vi "TRANSPOSED_VERTREAD_CSV_import_control_lasers_and_SMs_and_ICC4C_CAM_Trigger.vi"() -> ()   [LabVIEW 2021]
uses:
  <vilib>/DAQmx/write.llb/DAQmx Write (Analog 1D DBL NChan 1Samp).vi
  <vilib>/DAQmx/create/channels.llb/DAQmx Create Channel (AO-Voltage-Basic).vi
  <vilib>/Utility/file.llb/Read Delimited Spreadsheet (DBL).vi
  <vilib>/DAQmx/miscellaneous.llb/DAQmx Fill In Error Info.vi
panel:
  out "Raw  Inner Loop Iternation":dbl
  out "Numeric":dbl
  out "Trigger_Phase_Iterations":i32
  out "Cam_Trigger_Lo":dbl
  out "Cam_Trigger_Hi":dbl
  out "Sequence Length":i32
  in  "Delay (ADDS 50ms)":i32
  in  "ICC4C 3 (0-10V)":dbl
  in  "ICC4C 2 (0-10V)":dbl
  in  "ICC4C 1 (0-10V)":dbl
  in  "ICC4C 0 (0-10V)":dbl
  in  "Y2 (-10-10V)":dbl
  in  "X2 (-10-10V)":dbl
  in  "Continue Cycle?":bool
  out "Full Cycles":i32
  out "Mirror_Phase_Iterations":i32
  out "Y1 (-10-10V)":dbl format="%_6g"
  out "X1 (-10-10V)":dbl format="%_6g"
  in  "Blanking (0-10v)":dbl=10.0
  in  "561 (0-10v)":dbl
  in  "514 (0-10v)":dbl
  in  "488 (0-10v)":dbl
  in  "445 (0-10v)":dbl
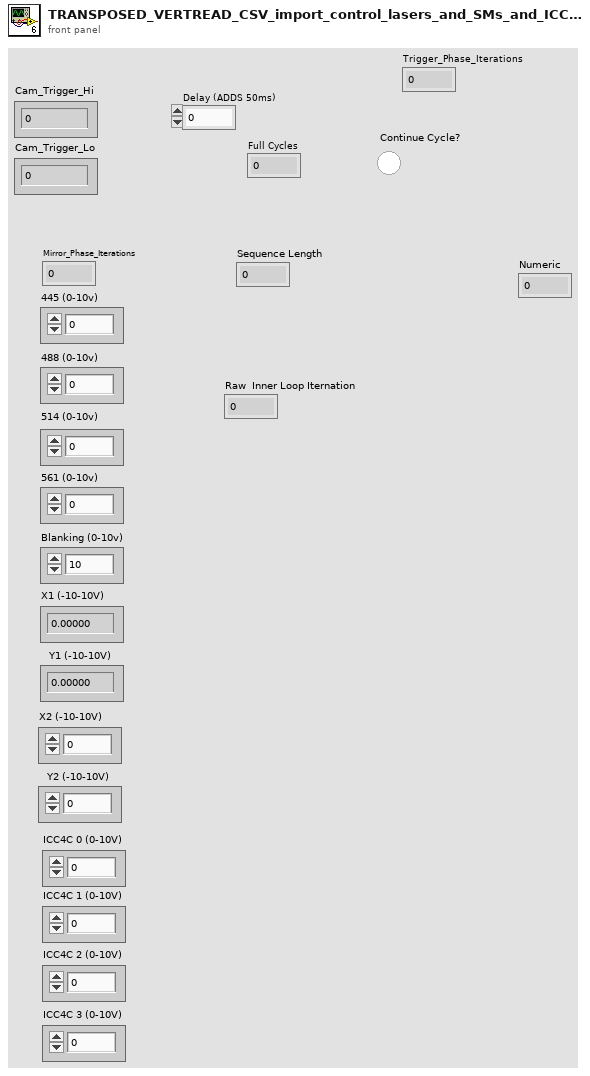
[diagram p1: front panel]
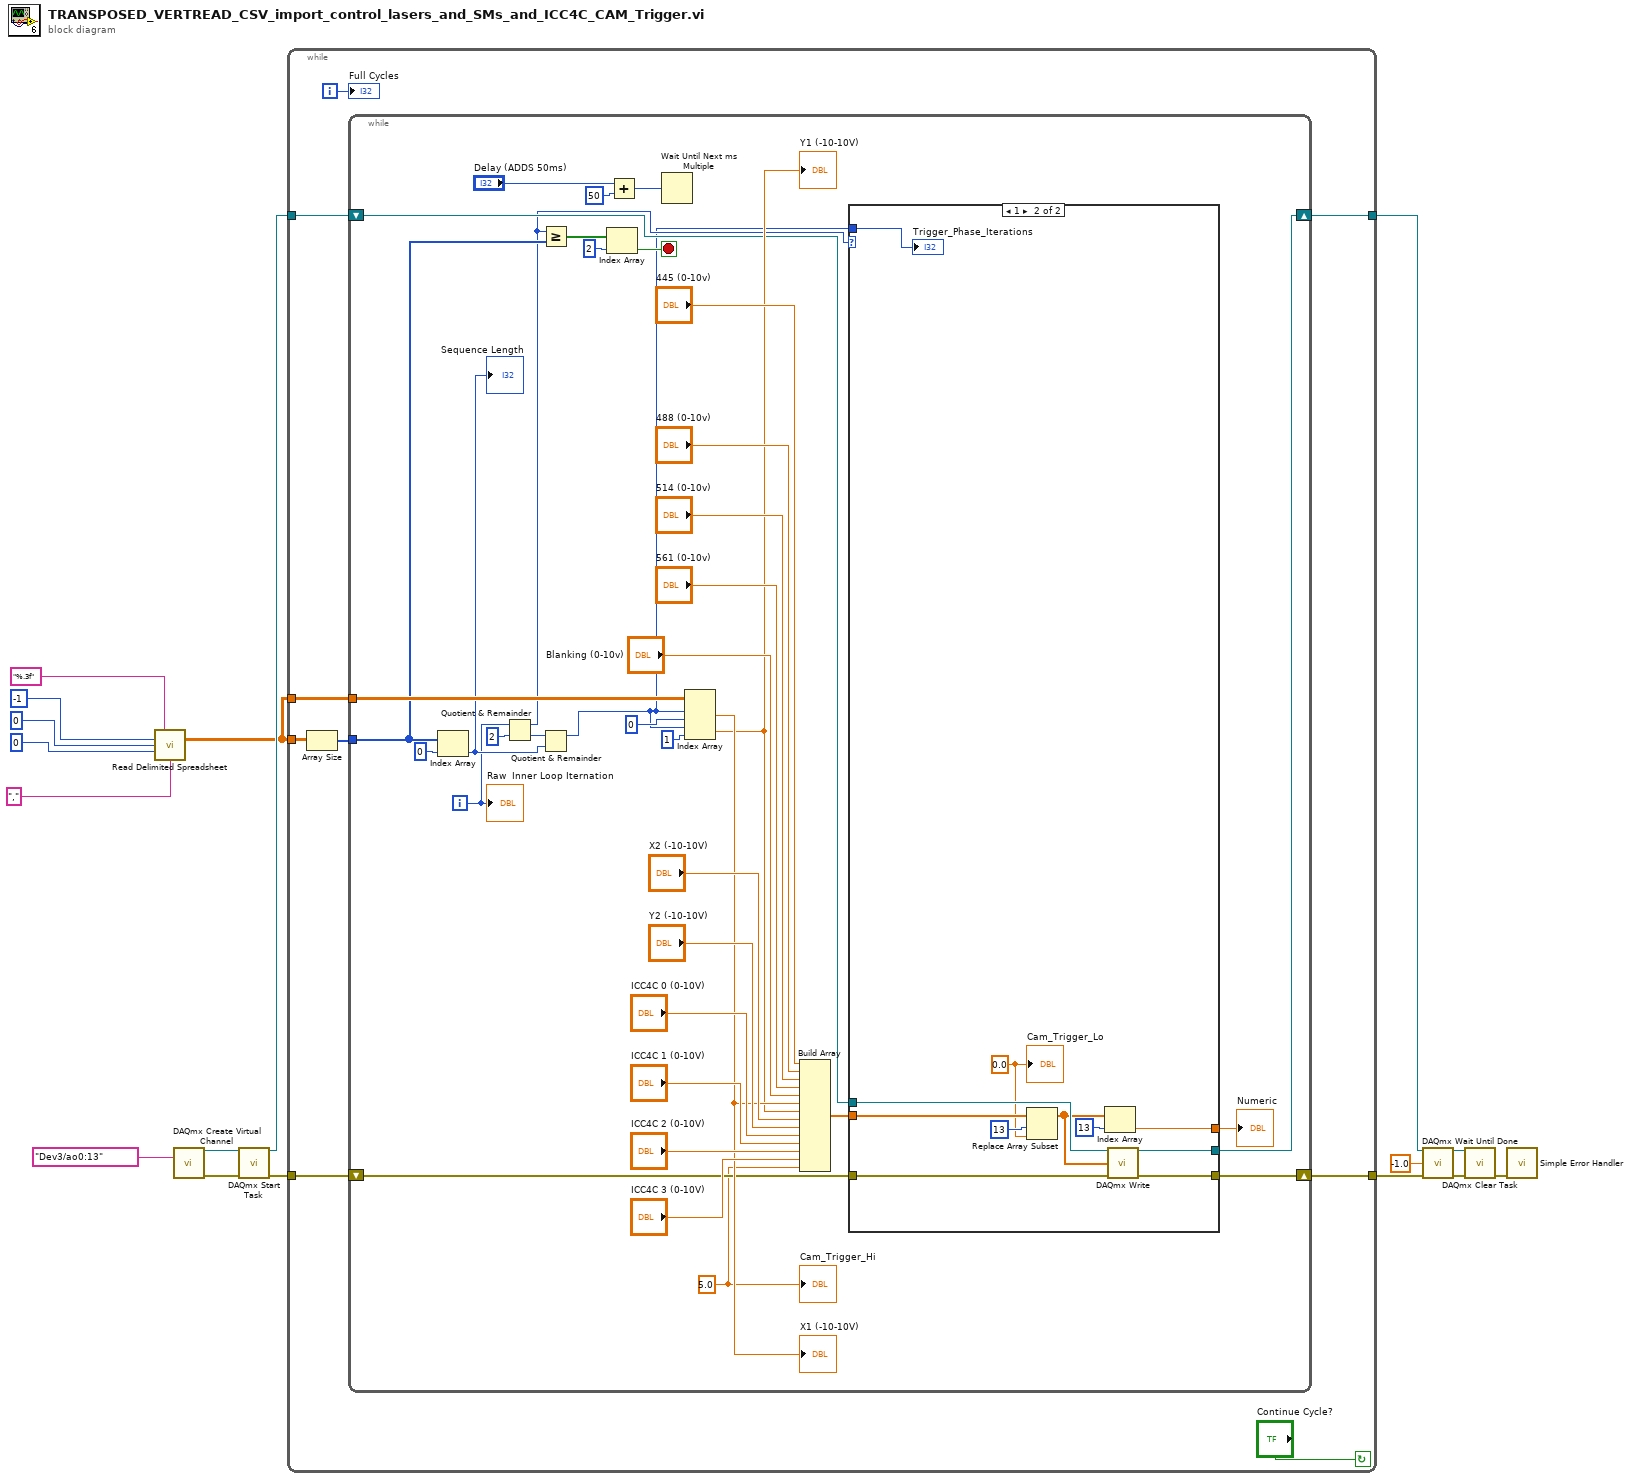
[diagram p0: block diagram]
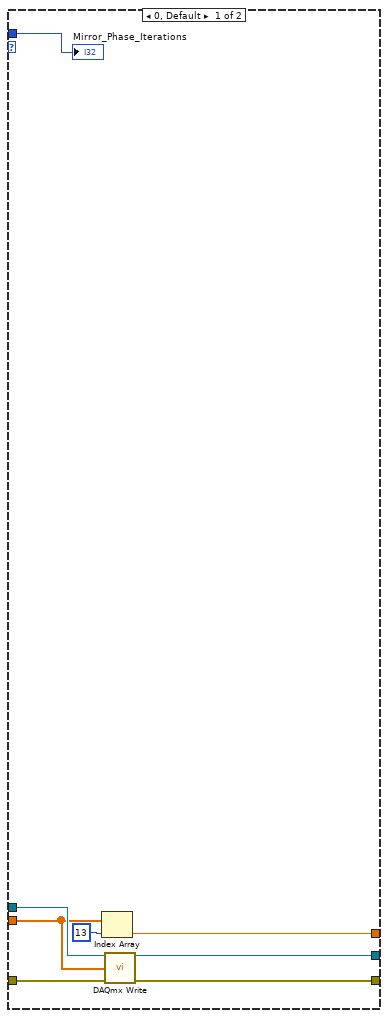
[diagram p2: hidden frame]
diagram:
  n1 = call-poly <vilib>:"Read Delimited Spreadsheet.vi"("format (%.3f)"="%.3f", "number of rows (all:-1)"=-1, "start of read offset (chars.:0)"=0, "max characters/row  (no limit:0)"=0, "delimiter (\\t)"=",") -> ("all rows"=w6:dbl[][])  [unwired: 5 in, 5 out]
  n2 = call-poly <vilib>:"DAQmx Create Virtual Channel.vi"("physical channels"=tag "Dev3/ao0:13") -> ("task out"=w10:refnum<k21>, "error out"=w9:errorcluster)  [unwired: 13 in]
  n3 = call <vilib>:"DAQmx Start Task.vi"("task/channels in"=w10, "error in"=w9) -> ("task out"=w8:refnum<k21>, "error out"=w7:errorcluster)  [unwired: 12 in]
  n4 = while {
    tunnel: [w23] -> w13
    tunnel: [w22] -> w12
    tunnel: w8 -> [w25]
    tunnel: w7 -> [w24]
    tunnel: w6 -> [w20]
    tunnel: w6 -> [w19]
    i -> [w26]
    stop <- "Continue Cycle?" continue-if-true
    n5 = Array Size(array=w20) -> (size(s)=w21:i32[])
    n6 = while {
      shift-right: [w41] -> w23
      shift-left: w25 -> [w39]
      shift-right: [w42] -> w22
      shift-left: w24 -> [w38]
      tunnel: w21 -> [w47]
      tunnel: w19 -> [w49]
      i -> [w35]
      stop <- w50 stop-if-true
      w27 = 5.0
      n7 = Index Array(array=w47, index=0) -> (element=w45:i32)
      "Sequence Length" <- w45
      n8 = Quotient & Remainder(x=w35, y=2) -> (x-y*floor(x/y)=w36:i32, floor(x/y)=w34:i32)
      n9 = Greater Or Equal?(x=w36, y=w47) -> (x >= y?=w51:bool[])
      n10 = Quotient & Remainder(x=w34, y=w45) -> (x-y*floor(x/y)=w28:i32)  [unwired: 1 out]
      n11 = Index Array(array=w51, index=2) -> (element=w50:bool)
      n12 = Add(x="Delay (ADDS 50ms)", y=50) -> (x+y=w31:i32)
      n13 = Wait Until Next ms Multiple(millisecond multiple=w31) -> ()  [unwired: 1 out]
      n14 = Index Array(array=w49, index (row) #1=w28, index (col) #1=0, index (row) #2=w28, index (col) #2=1) -> (element #1=w52:dbl, element #2=w48:dbl)
      "X1 (-10-10V)" <- w52
      "Y1 (-10-10V)" <- w48
      n15 = Build Array("445 (0-10v)", "488 (0-10v)", "514 (0-10v)", "561 (0-10v)", "Blanking (0-10v)", w52, w48, "X2 (-10-10V)", "Y2 (-10-10V)", "ICC4C 0 (0-10V)", "ICC4C 1 (0-10V)", "ICC4C 2 (0-10V)", "ICC4C 3 (0-10V)", w27) -> (w43:dbl[])
      n16 = case shown="1" w36 {
        tunnel: w39 -> [w71 w82]
        tunnel: [w68 w81] -> w41
        tunnel: w38 -> [w70 w80]
        tunnel: [w69 w76] -> w42
        tunnel: w43 -> [w67 w79]
        tunnel: w28 -> [w64 w77]
        tunnel: [w65 w73] -> w37
        frame 0, Default {
          n17 = Index Array(array=w67, index=13) -> (element=w65:dbl)
          n18 = call-poly <vilib>:"DAQmx Write.vi"("task/channels in"=w71, "data"=w67, "error in"=w70) -> ("task out"=w68:refnum<k21>, "error out"=w69:errorcluster)  [unwired: 10 in, 1 out]
          "Mirror_Phase_Iterations" <- w64
        }
        frame 1 {
          w72 = 0.0
          n19 = Replace Array Subset(array=w79, new element=w72, index=13) -> (w74:dbl[])
          n20 = Index Array(array=w74, index=13) -> (element=w73:dbl)
          n21 = call-poly <vilib>:"DAQmx Write.vi"("task/channels in"=w82, "data"=w74, "error in"=w80) -> ("task out"=w81:refnum<k21>, "error out"=w76:errorcluster)  [unwired: 10 in, 1 out]
          "Cam_Trigger_Lo" <- w72
          "Trigger_Phase_Iterations" <- w77
        }
      }
      "Numeric" <- w37
      "Cam_Trigger_Hi" <- w27
      "Raw  Inner Loop Iternation" <- w35
    }
    "Full Cycles" <- w26
  }
  n22 = call <vilib>:"DAQmx Wait Until Done.vi"("task/channels in"=w13, "timeout (sec)"=-1.0, "error in"=w12) -> ("task out"=w16:refnum<k21>, "error out"=w15:errorcluster)  [unwired: 11 in]
  n23 = call <vilib>:"DAQmx Clear Task.vi"("task in"=w16, "error in"=w15) -> ("error out"=w17:errorcluster)  [unwired: 13 in]
  n24 = call <vilib>:"Simple Error Handler.vi"("error in (no error)"=w17) -> ()  [unwired: 4 in, 5 out]
